vi "_SimpleDEMO.vi"() -> ()   [LabVIEW 2012]
panel:
  out "AutoLaunch?":bool
  out "ini file":string
  out "Main Directory":string
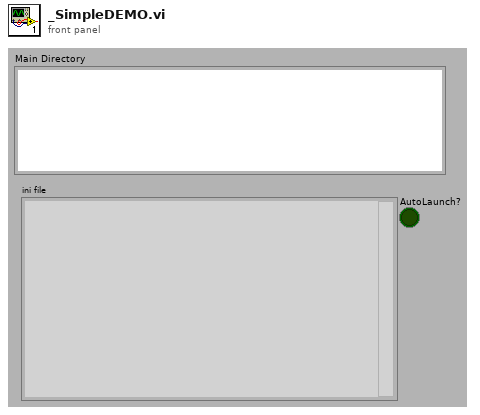
[diagram p1: front panel]
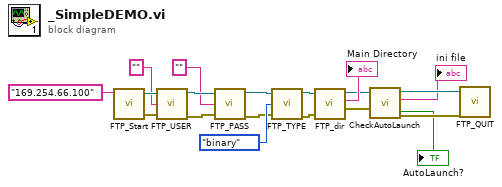
[diagram p0: block diagram]
diagram:
  n1 = call <userlib>:"FTP_Start.vi"("address"="169.254.66.100") -> ("connection ID"=w12:refnum<k5>, "error out"=w11:errorcluster)  [unwired: 4 in, 1 out]
  n2 = call <userlib>:"FTP_USER.vi"("connection ID"=w12, "user"="", "error out"=w11) -> ("connection ID out"=w14:refnum<k5>, "error out 2"=w13:errorcluster)  [unwired: 2 out]
  n3 = call <userlib>:"FTP_PASS.vi"("connection ID"=w14, "password"="", "error in"=w13) -> ("connection ID out"=w10:refnum<k5>, "error out"=w9:errorcluster)  [unwired: 2 out]
  n4 = call <userlib>:"FTP_TYPE.vi"("connection ID"=w10, "type (query)"=enum16{"(query)", "ASCII", "binary"}."binary", "error in"=w9) -> ("connection ID out"=w19:refnum<k5>, "error out"=w18:errorcluster)  [unwired: 2 out]
  n5 = call <userlib>:"FTP_dir.vi"("connection ID"=w19, "error in"=w18) -> ("connection ID out"=w6:refnum<k5>, "reply string"=→"Main Directory":string, "error out"=w5:errorcluster)  [unwired: 2 out]
  n6 = call <userlib>:"CheckAutoLaunch.vi"("connection ID in"=w6, 3:w5) -> ("AutoLaunch?"=→"AutoLaunch?":bool, "error out"=w4:errorcluster, "ini file"=→"ini file":string, "connection ID out"=w3:refnum<k5>)  [unwired: 1 in, 1 out]
  n7 = call <userlib>:"FTP_QUIT.vi"("connection ID"=w3, "error in"=w4) -> ()  [unwired: 4 out]
